vi "3201告警信息改变发送 (子VI).vi"(8 "错误输入":errorcluster caption="错误输出") -> (0 "错误输出":errorcluster)   [LabVIEW 2016, in "数据传输系统-04.lvlib"]
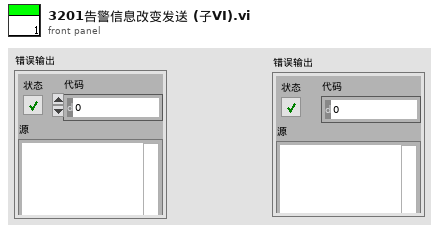
[diagram p1: front panel]
types:
  T1 = cluster{"温度告警":u16, "湿度告警":u16, "烟感告警":u16, "水浸告警":u16, "门禁告警":u16, "超标留样瓶满告警":u16}
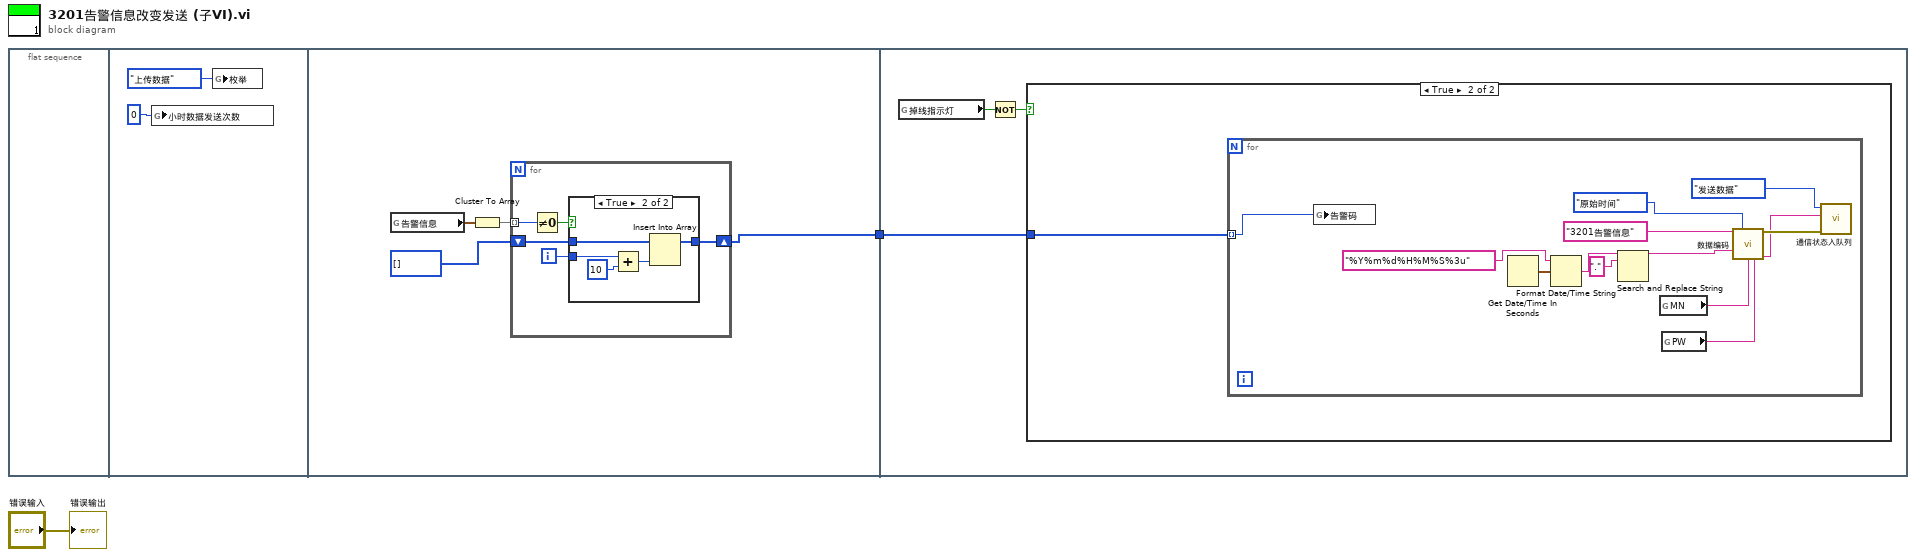
[diagram p0: block diagram]
diagram:
  n1 = flat-sequence {
    tunnel: [w6] -> w1
    tunnel: w1 -> [w20]
    frame #0 {
    }
    frame #1 {
      n2 = global write "全局 小时数据发送次数.vi" "小时数据发送次数"(0 ("小时数据发送次数")) -> ()
      n3 = global write "全局1.vi" "枚举"(enum16{"返回请求应答", "上传数据", "返回执行结果"}."上传数据" ("枚举")) -> ()
    }
    frame #2 {
      n4 = global read "全局1.vi" "告警信息"() -> (w8:T1)
      n5 = Cluster To Array(cluster=w8) -> (array=w7:u16[])
      n6 = for {
        tunnel: w7 -> [w13] mode=indexing
        shift-right: [w9] -> w6
        shift-left: i32[] [] -> [w10]
        i -> [w12]
        n7 = Not Equal To 0?(x=w13) -> (x != 0?=w11:bool)
        n8 = case shown="True" w11 {
          tunnel: w12 -> [_ w17]
          tunnel: w10 -> [w14 w19]
          tunnel: [w14 w18] -> w9
          frame False {
          }
          frame True {
            n9 = Add(x=w17, y=10) -> (x+y=w15:i32)
            n10 = Insert Into Array(array=w19, new element=w15) -> (w18:i32[])  [unwired: 1 in]
          }
        }
      }
    }
    frame #3 {
      n11 = global read "全局 数据发送重叠.vi" "掉线指示灯"() -> (w22:bool)
      n12 = Not(x=w22) -> (.not. x?=w21:bool)
      n13 = case shown="True" w21 {
        tunnel: w20 -> [_ w23]
        frame False {
        }
        frame True {
          n14 = for {
            tunnel: w23 -> [w24] mode=indexing
            n15 = global write "全局 小时数据发送次数.vi" "告警码"(w24) -> ()
            n16 = Get Date/Time In Seconds() -> (seconds since 1Jan1904=w34:timestamp)
            n17 = Format Date/Time String(time format string (%c)="%Y%m%d%H%M%S%3u" ("时间格式字符串(%c)"), seconds (now)=w34) -> (date/time string=w33:string)  [unwired: 1 in]
            n18 = Search and Replace String(input string=w33, search string="." ("搜索字符串")) -> (result string=w31:string)  [unwired: 6 in, 3 out]
            n19 = global read "断电保存全局.vi" "MN"() -> (w30:string)
            n20 = global read "断电保存全局.vi" "PW"() -> (w29:string)
            n21 = call "数据编码.vi"("table输入"="3201告警信息" ("新元素/子数组"), "仪器参数上传时间"=enum16{"精确到小时", "原始时间"}."原始时间", "QN"=w31, "MN"=w30, "PW"=w29) -> ("错误常量"=w28:errorcluster, "通讯包字符串"=w25:string)  [unwired: 9 in]
            n22 = call "通信状态入队列.vi"("错误输入（无错误）"=w28, "发送报文"=w25, "枚举"=enum16{"打开连接", "发送数据", "读取数据", "数据处理", "关闭连接"}."发送数据") -> ()  [unwired: 8 in, 1 out]
          }
        }
      }
    }
  }
  "错误输出" <- "错误输入"
